vi "getTimingsUsed.vi"(8 "error in (no error)":errorcluster, 11 "CameraSettingsManager.lvclass in":refnum<class "CameraSettingsManager.lvclass">) -> (0 "error out":errorcluster, 2 "Timings Used":T1, 3 "CameraSettingsManager.lvclass out":refnum<class "CameraSettingsManager.lvclass">)   [LabVIEW 2011, in "Tools.lvlib" / "Settings.lvlib" / "CameraSettingsManager.lvclass"]
uses:
  CameraSettingsManager.lvclass
  CameraSettingsManager.lvclass/CameraSettingsManager.ctl
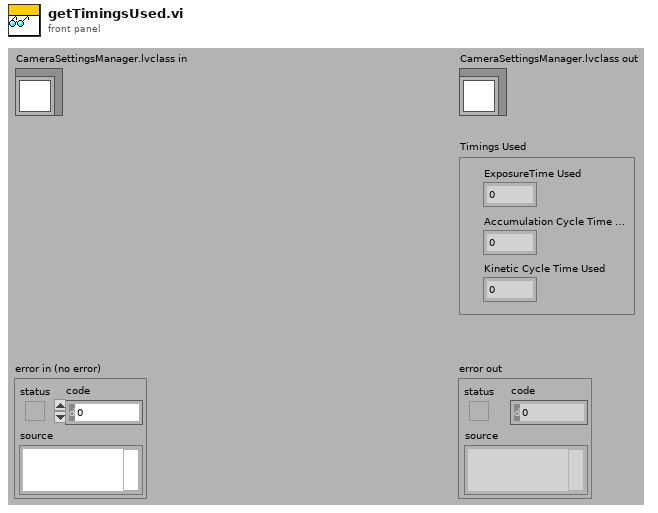
[diagram p1: front panel]
types:
  T1 = cluster{"ExposureTime Used":dbl, "Accumulation Cycle Time Used":dbl, "Kinetic Cycle Time Used":dbl}
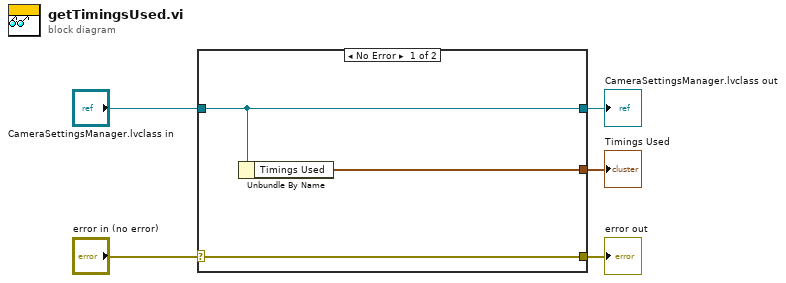
[diagram p0: block diagram]
diagram:
  n1 = case shown="No Error" "error in (no error)" {
    selector: "error in (no error)" -> [w8 w9]
    tunnel: [w8 w9] -> w4
    tunnel: [w7 w10] -> w2
    tunnel: "CameraSettingsManager.lvclass in" -> [w7 w10]
    tunnel: [w6 _] -> w1
    frame No Error {
      n2 = Unbundle By Name(w7) -> ("Timings Used"=w6:T1)
    }
    frame Error {
    }
  }
  "error out" <- w4
  "CameraSettingsManager.lvclass out" <- w2
  "Timings Used" <- w1
